vi "Write Laser Lines File.vi"() -> ()   [LabVIEW 2016]
uses:
  MC AOTF Controls/MC AOTF Lines Lines Control.ctl
panel:
  in  "Laser Lines":T1
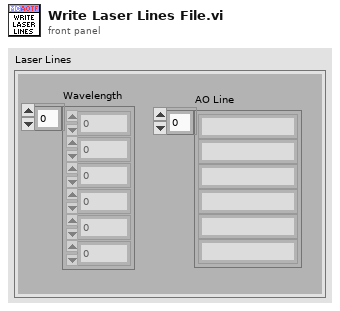
[diagram p1: front panel]
types:
  T1 = typedef "MC AOTF Lines Lines Control.ctl" = cluster{"Wavelength":u16[], "AO Line":string[]}
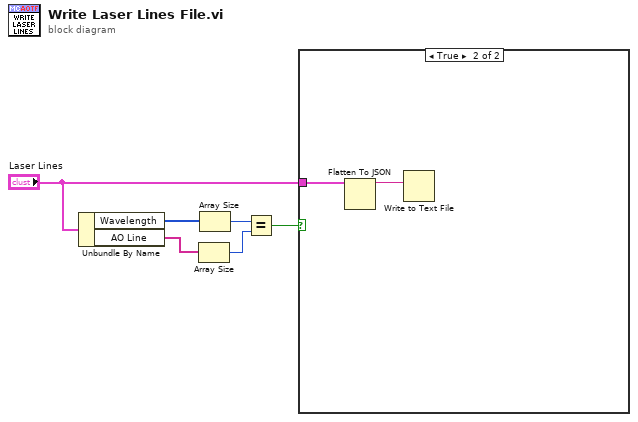
[diagram p0: block diagram]
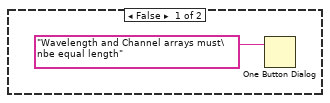
[diagram p2: hidden frame]
diagram:
  n1 = Unbundle By Name("Laser Lines") -> ("Wavelength"=w6:u16[], "AO Line"=w5:string[])
  n2 = Array Size(array=w5) -> (size(s)=w3:i32)
  n3 = Array Size(array=w6) -> (size(s)=w4:i32)
  n4 = Equal?(x=w4, y=w3) -> (x = y?=w2:bool)
  n5 = case shown="True" w2 {
    tunnel: "Laser Lines" -> [_ w9]
    frame False {
      n6 = One Button Dialog(message="Wavelength and Channel arrays must\nbe equal length") -> ()  [unwired: 1 in, 1 out]
    }
    frame True {
      n7 = Flatten To JSON(anything=w9) -> (JSON string=w8:string)  [unwired: 2 in, 1 out]
      n8 = Write to Text File(text=w8) -> ()  [unwired: 3 in, 3 out]
    }
  }
